vi "Perform Full Scale Error Measurement.vi"(7 "Measurement Context":refnum<class "MeasurementContext.lvclass">, 8 "error in":errorcluster, 9 "Sweep transition settings":T4, 10 "device sessions":T2, 11 "measurement configuration":T5={"Input channel"=1, "Full scale range"=10.0, "Transition span"=1.5, "Transition step size"=0.05, "Analog source resource name"="", "Digital capture resource name"="", "Digital capture sample rate"=800000.0, "Digital capture samples"=10000, "DMM resource name"="", "DMM range"=10.0, "DMM resolution"=5.5} {"DMM range" format="%#_6pV"; "Digital capture sample rate" format="%#_6pS/s"; "Transition step size" format="%#_gLSB"; "Transition span" format="%#_gLSB"; "Full scale range" format="%#_6pV"}) -> (0 "error out":errorcluster, 2 "measurement results out":T3)   [LabVIEW 2021, in "adc_fullScaleError.lvlib"]
uses:
  adc_fullScaleError.lvlib
  Measurement Configuration.ctl
  Controls/Sweep Transition Settings.ctl
  Measurement Results.ctl
  <vilib>/MeasurementLink/MeasurementLink Measurement Server/Classes/MeasurementContext/MeasurementContext.lvclass
  <vilib>/gRPC/LabVIEW gRPC Library/Shared/grpcId.ctl
  <vilib>/Analysis/1siggen.llb/Ramp Pattern by Samples.vi
  <vilib>/DAQmx/write.llb/DAQmx Write (Analog 1D DBL 1Chan NSamp).vi
  <instrlib>/niDMM/nidmm.llb/niDMM Configure Measurement Digits.vi
  <vilib>/MeasurementLink/MeasurementLink Measurement Server/Classes/MeasurementContext/Accessor/Is Canceled.vi
  <vilib>/DAQmx/miscellaneous.llb/DAQmx Fill In Error Info.vi
  <vilib>/Analysis/baseanly.llb/Unimode.vi
  <vilib>/Analysis/NI_AALBase.lvlib
  shared/digitalInterface/client/dcvmDPI_AD7606B_clientImpl/dcvmDPI_AD7606B_clientImpl.lvlib
  <vilib>/gRPC/LabVIEW gRPC Library/grpc-lvsupport-release.lvlib
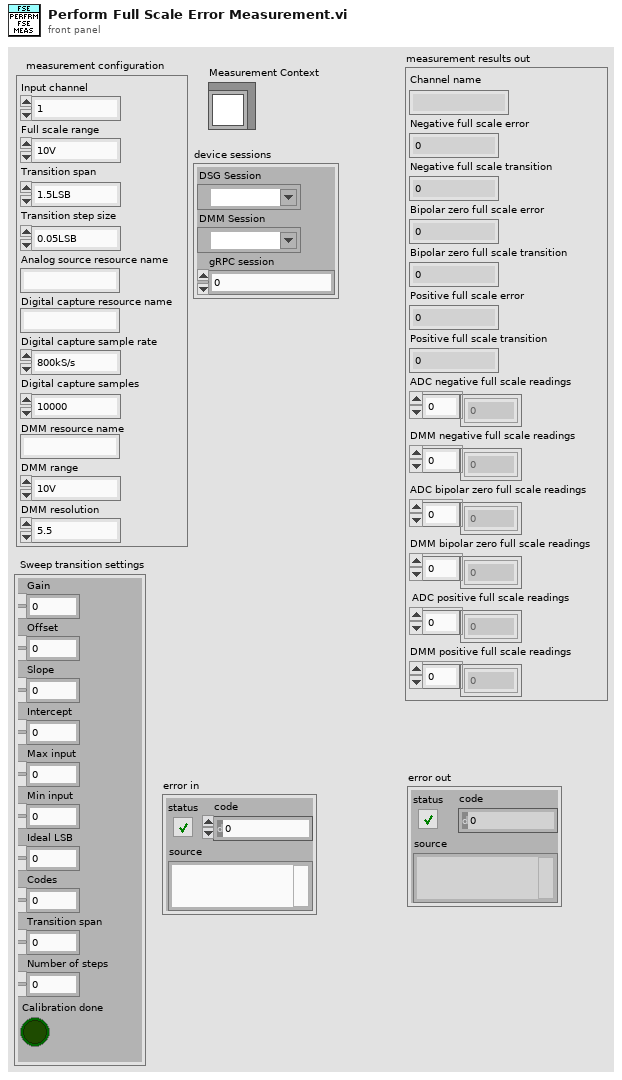
[diagram p1: front panel]
types:
  T1 = typedef "grpc-lvsupport-release.lvlib/grpcId.ctl" = u64
  T2 = cluster{"DSG Session":refnum<k21>, "DMM Session":refnum<k15>, "gRPC session":T1}
  T3 = typedef "adc_fullScaleError.lvlib/Measurement Results.ctl" = cluster{"Channel name":string, "Negative full scale error":dbl, "Negative full scale transition":dbl, "Bipolar zero full scale error":dbl, "Bipolar zero full scale transition":dbl, "Positive full scale error":dbl, "Positive full scale transition":dbl, "ADC negative full scale readings":dbl[], "DMM negative full scale readings":dbl[], "ADC bipolar zero full scale readings":dbl[], "DMM bipolar zero full scale readings":dbl[], "ADC positive full scale readings":dbl[], "DMM positive full scale readings":dbl[]}
  T4 = typedef "adc_fullScaleError.lvlib/Sweep Transition Settings.ctl" = cluster{"Gain":dbl, "Offset":dbl, "Slope":dbl, "Intercept":dbl, "Max input":dbl, "Min input":dbl, "Ideal LSB":dbl, "Codes":dbl, "Transition span ":dbl, "Number of steps":i32, "Calibration done":bool}
  T5 = typedef "adc_fullScaleError.lvlib/Measurement Configuration.ctl" = cluster{"Input channel":i32, "Full scale range":dbl, "Transition span":dbl, "Transition step size":dbl, "Analog source resource name":string, "Digital capture resource name":string, "Digital capture sample rate":dbl, "Digital capture samples":u32, "DMM resource name":string, "DMM range":dbl, "DMM resolution":dbl}
  T6 = typedef "adc_fullScaleError.lvlib/Sweep Configurations.ctl" = cluster{"Start":dbl, "Stop":dbl, "Number of steps":i32}
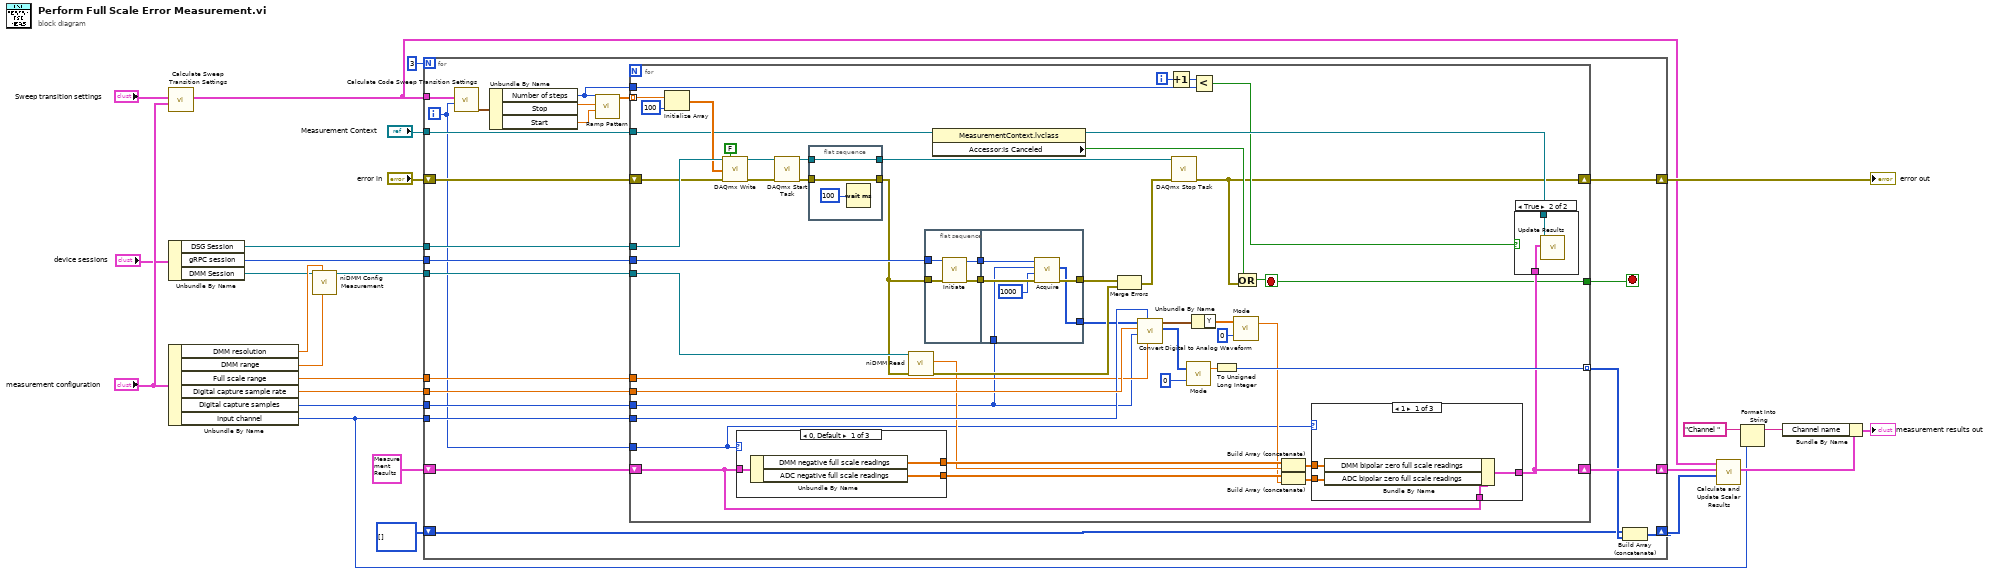
[diagram p0: block diagram]
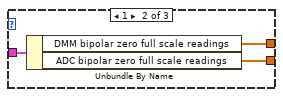
[diagram p2: hidden frame]
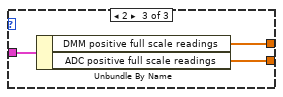
[diagram p3: hidden frame]
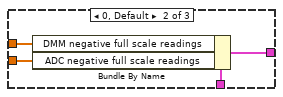
[diagram p5: hidden frame]
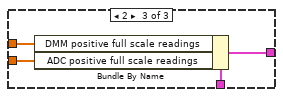
[diagram p6: hidden frame]
diagram:
  n1 = call "Calculate Sweep Transition Settings.vi"("measurement configuration"="measurement configuration", "Sweep Transition Settings In"="Sweep transition settings") -> ("Sweep Transition Settings Out"=w2:T4)  [unwired: 9 in]
  n2 = Unbundle By Name("device sessions") -> ("DSG Session"=w26:refnum<k21>, "gRPC session"=w25:T1, "DMM Session"=w12:refnum<k15>)
  n3 = Unbundle By Name("measurement configuration") -> ("DMM resolution"=w16:dbl, "DMM range"=w15:dbl, "Full scale range"=w14:dbl, "Digital capture sample rate"=w24:dbl, "Digital capture samples"=w23:u32, "Input channel"=w5:i32)
  n4 = call-poly <instrlib>:"niDMM Config Measurement.vi"("Range"=w15, "Resolution in Digits"=w16, "instrument handle"=w12) -> ("instrument handle out"=w17:refnum<k15>)  [unwired: 7 in, 1 out]
  n5 = for {
    N: 3 -> [_]
    tunnel: w2 -> [w46]
    tunnel: w26 -> [w44]
    tunnel: w25 -> [w43]
    tunnel: w17 -> [w42]
    tunnel: w24 -> [w41]
    tunnel: w23 -> [w40]
    tunnel: w5 -> [w39]
    shift-right: [w34] -> w19
    shift-left: "error in" -> [w38]
    shift-right: [w32] -> w8
    shift-left: T3 {"Channel name"="", "Negative full scale error"=0.0, "Negative full scale transition"=0.0, "Bipolar zero full scale error"=0.0, "Bipolar zero full scale transition"=0.0, "Positive full scale error"=0.0, "Positive full scale transition"=0.0, "ADC negative full scale readings"=[], "DMM negative full scale readings"=[], "ADC bipolar zero full scale readings"=[], "DMM bipolar zero full scale readings"=[], "ADC positive full scale readings"=[], "DMM positive full scale readings"=[]} ("measurement results") -> [w36]
    tunnel: w14 -> [w37]
    tunnel: "Measurement Context" -> [w35]
    shift-right: [w30] -> w9
    shift-left: u32[][] [] -> [w29]
    i -> [w28]
    stop <- w27 stop-if-true
    n6 = call "Calculate Code Sweep Transition Settings.vi"("Code transition type"=w28, "Sweep transition settings"=w46) -> ("Sweep configurations"=w49:T6)  [unwired: 6 in, 3 out]
    n7 = Unbundle By Name(w49) -> ("Number of steps"=w33:i32, "Stop"=w48:dbl, "Start"=w47:dbl)
    n8 = call-poly <vilib>:"Ramp Pattern.vi"("start"=w47, "end"=w48, "samples"=w33) -> ("Ramp Pattern"=w45:dbl[])  [unwired: 7 in, 1 out]
    n9 = for {
      tunnel: w45 -> [w98] mode=indexing
      tunnel: w41 -> [w88]
      tunnel: w40 -> [w52]
      shift-right: [w58] -> w34
      shift-left: w38 -> [w84]
      tunnel: [w77] -> w31 mode=indexing
      tunnel: w39 -> [w83]
      tunnel: w37 -> [w76]
      tunnel: w44 -> [w96]
      tunnel: w43 -> [w56]
      tunnel: w42 -> [w89]
      shift-right: [w59] -> w32
      shift-left: w36 -> [w70]
      tunnel: w28 -> [w71]
      tunnel: w35 -> [w66]
      tunnel: w33 -> [w62]
      tunnel: [w57] -> w27
      i -> [w64]
      stop <- w57 stop-if-true
      n10 = Initialize Array(w98, 100 ("dimension size")) -> (w90:dbl[])
      n11 = call-poly <vilib>:"DAQmx Write.vi"("task/channels in"=w96, "auto start"=FALSE, "data"=w90, "error in"=w84) -> ("task out"=w94:refnum<k21>, "error out"=w93:errorcluster)  [unwired: 9 in, 1 out]
      n12 = case shown="0, Default" w71 {
        tunnel: w70 -> [w111 w114 w117]
        tunnel: [w110 w113 w116] -> w75
        tunnel: [w109 w112 w115] -> w74
        frame 0, Default {
          n13 = Unbundle By Name(w111) -> ("DMM negative full scale readings"=w110:dbl[], "ADC negative full scale readings"=w109:dbl[])
        }
        frame 1 {
          n14 = Unbundle By Name(w114) -> ("DMM bipolar zero full scale readings"=w113:dbl[], "ADC bipolar zero full scale readings"=w112:dbl[])
        }
        frame 2 {
          n15 = Unbundle By Name(w117) -> ("DMM positive full scale readings"=w116:dbl[], "ADC positive full scale readings"=w115:dbl[])
        }
      }
      n16 = call <vilib>:"DAQmx Start Task.vi"("task/channels in"=w94, "error in"=w93) -> ("task out"=w91:refnum<k21>, "error out"=w92:errorcluster)  [unwired: 12 in]
      n17 = flat-sequence {
        tunnel: w92 -> [w118]
        tunnel: w91 -> [w119]
        tunnel: [w119] -> w85
        tunnel: [w118] -> w55
        frame #0 {
          n18 = Wait (ms)(milliseconds to wait=u32 100) -> ()  [unwired: 1 out]
        }
      }
      n19 = call <instrlib>:"niDMM Read.vi"("error in (no error)"=w55, "instrument handle"=w89) -> ("error out"=w86:errorcluster, "Measurement"=w73:dbl)  [unwired: 7 in, 1 out]
      n20 = flat-sequence {
        tunnel: w56 -> [w102]
        tunnel: w55 -> [w101]
        tunnel: [w100] -> w54
        tunnel: [w99] -> w53
        tunnel: w54 -> [w108]
        tunnel: w53 -> [w107]
        tunnel: w52 -> [w106]
        tunnel: [w104] -> w51
        tunnel: [w103] -> w50
        frame #0 {
          n21 = call "Initiate.vi"("error in"=w101, "gRPC session in"=w102) -> ("error out"=w99:errorcluster, "gRPC session out"=w100:T1)  [unwired: 8 in]
        }
        frame #1 {
          n22 = call "Acquire.vi"("error in"=w107, "Timeout (ms)"=1000, "Digital capture samples"=w106, "gRPC session in"=w108) -> ("error out"=w104:errorcluster, "Digital waveform"=w103:u32[])  [unwired: 5 in, 1 out]
        }
      }
      n23 = property class="MeasurementContext.lvclass"(reference=w66) -> (reference out=w61:refnum<class "MeasurementContext.lvclass">, "Accessor:Is Canceled"=w65:bool)  [unwired: 1 in, 1 out]
      n24 = Merge Errors(w51, w86) -> (w67:errorcluster)
      n25 = call "Convert Digital to Analog Waveform.vi"("full scale range"=w76, "channel index"=w83, "Number of samples"=w52, "Sample rate"=w88, "Digital waveform in"=w50) -> ("Digital waveform out"=w81:u32[], "Waveform"=w87:waveform(dbl))  [unwired: 4 in, 1 out]
      n26 = Increment(x=w64) -> (x+1=w63:i32)
      n27 = call <vilib>:"DAQmx Stop Task.vi"("task/channels in"=w85, "error in"=w67) -> ("error out"=w58:errorcluster)  [unwired: 12 in, 1 out]
      n28 = call-poly <vilib>:"Mode.vi"("intervals"=0, "X"=w81) -> ("mode"=w78:dbl)  [unwired: 1 out]
      n29 = Less?(x=w63, y=w62) -> (x < y?=w60:bool)
      n30 = Unbundle By Name(w87) -> ("Y"=w82:dbl[])
      n31 = To Unsigned Long Integer(number=w78) -> (unsigned 32bit integer=w77:u32)
      n32 = call-poly <vilib>:"Mode.vi"("intervals"=0, "X"=w82) -> ("mode"=w72:dbl)  [unwired: 1 out]
      n33 = Compound Arithmetic op=OR(w65, w58) -> (w57:bool)
      n34 = Build Array (concatenate)(w75, w73) -> (w69:dbl[])
      n35 = Build Array (concatenate)(w74, w72) -> (w68:dbl[])
      n36 = case shown="1" w71 {
        tunnel: w70 -> [w126 w130 w134]
        tunnel: w69 -> [w125 w129 w133]
        tunnel: w68 -> [w124 w128 w132]
        tunnel: [w123 w127 w131] -> w59
        frame 1 {
          n37 = Bundle By Name(cluster=w126, "DMM bipolar zero full scale readings"=w125, "ADC bipolar zero full scale readings"=w124) -> (w123:T3)
        }
        frame 0, Default {
          n38 = Bundle By Name(cluster=w130, "DMM negative full scale readings"=w129, "ADC negative full scale readings"=w128) -> (w127:T3)
        }
        frame 2 {
          n39 = Bundle By Name(cluster=w134, "DMM positive full scale readings"=w133, "ADC positive full scale readings"=w132) -> (w131:T3)
        }
      }
      n40 = case shown="True" w60 {
        tunnel: w61 -> [_ w122]
        tunnel: w59 -> [_ w121]
        frame False {
        }
        frame True {
          n41 = call <vilib>:"Update Results.vi"("Measurement Results"=w121, "MeasurementContext in"=w122) -> ()  [unwired: 8 in, 2 out]
        }
      }
    }
    n42 = Build Array (concatenate)(w29, w31) -> (w30:u32[][])
  }
  "error out" <- w19
  n43 = call "Calculate and Update Scalar Results.vi"("ADC codes"=w9, "measurement results"=w8, "Sweep transition settings"=w2) -> ("measurement results out"=w7:T3)  [unwired: 8 in]
  n44 = Format Into String(initial string="Channel ", w5) -> (resulting string=w21:string)  [unwired: 2 in, 1 out]
  n45 = Bundle By Name(cluster=w7, "Channel name"=w21) -> (→"measurement results out":T3)
